vi "Addressing_SearchAddress.vi"(7 "device_handle":i32, 8 "error in (no error)":errorcluster, 11 "Command":T1="SEARCHADDRH") -> (0 "error out":errorcluster)   [LabVIEW 2014, in "Driver_interaction.lvlib" / "Dali_usb_tridonics.lvclass"]
doc: "Get Address.\nSelect address type: ADDRH,ADDRM,ADDRL\nand start with data = 80 until get the correct value."
uses:
  Dali_usb_tridonics.lvclass
  Controls/Commands enum.ctl
  Vendor/Controls/Addressing_type.ctl
  Vendor/Dali_usb.lvlib
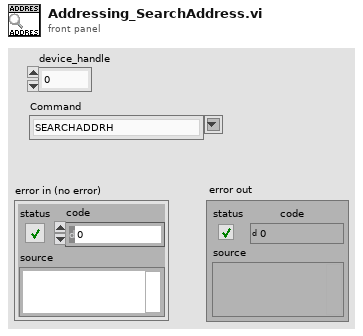
[diagram p1: front panel]
types:
  T1 = typedef "Driver_interaction.lvlib/Dali_usb_tridonics.lvclass/Commands enum.ctl" = string
  T2 = typedef "Dali_usb.lvlib/Addressing_type.ctl" = string
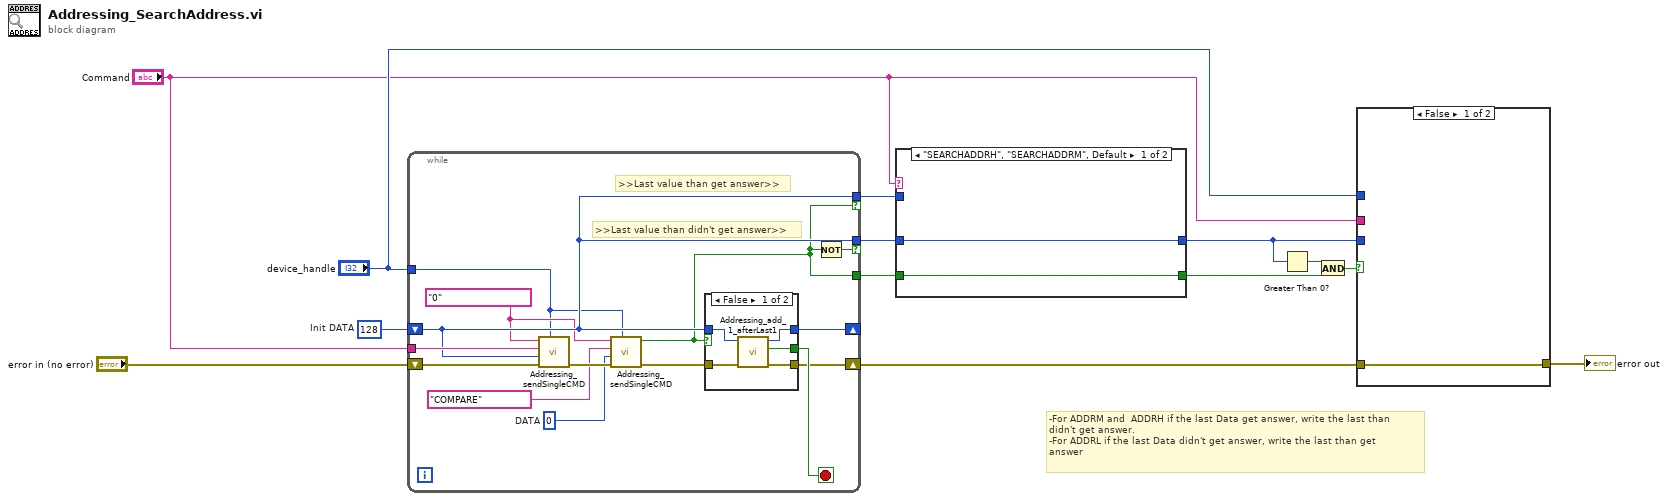
[diagram p0: block diagram]
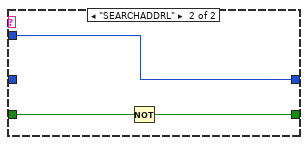
[diagram p2: hidden frame]
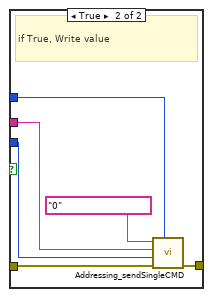
[diagram p3: hidden frame]
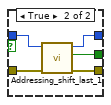
[diagram p4: hidden frame]
diagram:
  w13 = u32 128  # Init DATA
  # "-For ADDRM and  ADDRH if the last Data get answer, write the last than\ndidn't get answer.\n-For ADDRL if the last Data didn't get answer, write the last than get \nanswer"
  n1 = while {
    shift-right: [w27] -> _
    shift-left: w13 -> [w22]
    tunnel: [w22] -> w12 if=w25
    tunnel: [w16] -> w10
    tunnel: [w22] -> w11 if=w16
    tunnel: "Command" -> [w23]
    tunnel: "device_handle" -> [w19]
    shift-right: [w14] -> w8
    shift-left: "error in (no error)" -> [w24]
    stop <- w26 stop-if-true
    w17 = u32 0  # DATA
    w20 = T2 "0" ("addressing_type")
    # ">>Last value than didn't get answer>>"
    # ">>Last value than get answer>>"
    n2 = call "Addressing_sendSingleCMD.vi"("device_handle"=w19, "error in (no error)"=w24, "DATA"=w22, "Command"=w23, "addressing_type"=w20) -> ("error out"=w21:errorcluster)  [unwired: 5 in, 1 out]
    n3 = call "Addressing_sendSingleCMD.vi"("device_handle"=w19, "error in (no error)"=w21, "DATA"=w17, "Command"=T1 "COMPARE", "addressing_type"=w20) -> ("error out"=w15:errorcluster, "Answer Received?"=w16:bool)  [unwired: 5 in]
    n4 = case shown="False" w16 {
      tunnel: w22 -> [w32 w37]
      tunnel: [w31 w36] -> w27
      tunnel: [w30 w35] -> w26
      tunnel: w15 -> [w29 w34]
      tunnel: [w28 w33] -> w14
      frame False {
        n5 = call "Addressing_add_1_afterLast1.vi"("error in (no error)"=w29, "VALUE"=w32) -> ("error out"=w28:errorcluster, "Last value"=w30:bool, "Value + next 1"=w31:u32)  [unwired: 7 in]
      }
      frame True {
        n6 = call "Addressing_shift_last_1.vi"("error in (no error)"=w34, "VALUE"=w37) -> ("error out"=w33:errorcluster, "Last Value"=w35:bool, "Value >>1"=w36:u32)  [unwired: 7 in]
      }
    }
    n7 = Not(x=w16) -> (.not. x?=w25:bool)
  }
  n8 = case shown="\"SEARCHADDRH\", \"SEARCHADDRM\", Default" "Command" {
    tunnel: w12 -> [w39 _]
    tunnel: w11 -> [_ w42]
    tunnel: w10 -> [w38 w41]
    tunnel: [w38 w40] -> w2
    tunnel: [w39 w42] -> w4
    frame "SEARCHADDRH", "SEARCHADDRM", Default {
    }
    frame "SEARCHADDRL" {
      n9 = Not(x=w41) -> (.not. x?=w40:bool)
    }
  }
  n10 = Greater Than 0?(x=w4) -> (x > 0?=w3:bool)
  n11 = And(x=w3, y=w2) -> (x .and. y?=w1:bool)
  n12 = case shown="False" w1 {
    tunnel: "Command" -> [_ w49]
    tunnel: w4 -> [_ w48]
    tunnel: w8 -> [w43 w47]
    tunnel: [w43 w46] -> w7
    tunnel: "device_handle" -> [_ w45]
    frame False {
    }
    frame True {
      # "if True, Write value"
      n13 = call "Addressing_sendSingleCMD.vi"("device_handle"=w45, "error in (no error)"=w47, "DATA"=w48, "Command"=w49, "addressing_type"=T2 "0") -> ("error out"=w46:errorcluster)  [unwired: 5 in, 1 out]
    }
  }
  "error out" <- w7
